vi "Actor Template-Core_Process.vi"(0 "FTW Actor Instance Configuration":string="{\n  \"Identity\": \"ActorName\",\n  \"InboxAddress\": \"tcp://127.0.0.1:*\",\n  \"PublisherAddress\": \"tcp://127.0.0.1:*\",\n  \"DebugEnableInboxLogging\": false,\n  \"DebugEnableJobLogging\": false,\n  \"DebugShowPanel\": false\n}", 11 "ErrorIn":errorcluster) -> (15 "Error":errorcluster)   [LabVIEW 2013, in "Actor Template-Core.lvclass"]
uses:
  Actor Template-Core.lvclass
  src/Instance/FTW-ActorInstance.lvclass
  src/Message/Request/FTW-Message-IncomingRequest.lvclass
panel:
  # "#TODO\nhide controls for a GUI"
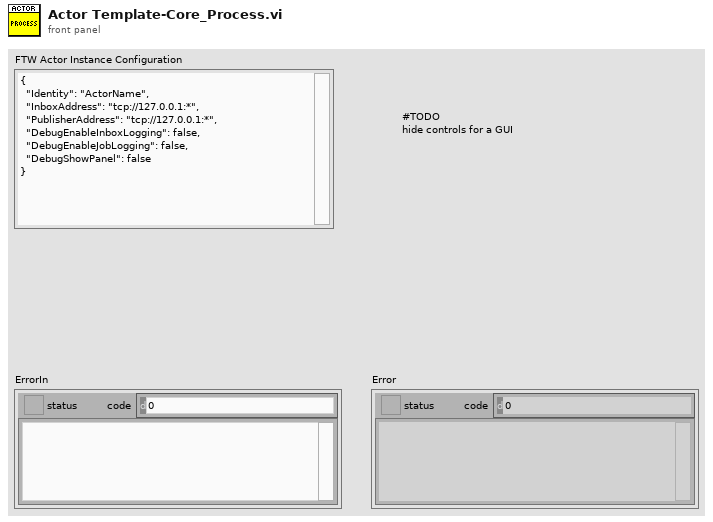
[diagram p1: front panel]
types:
  T1 = cluster{"Incoming Requests":refnum<event-registration>, "Additional Registration Types":refnum<event-registration>}
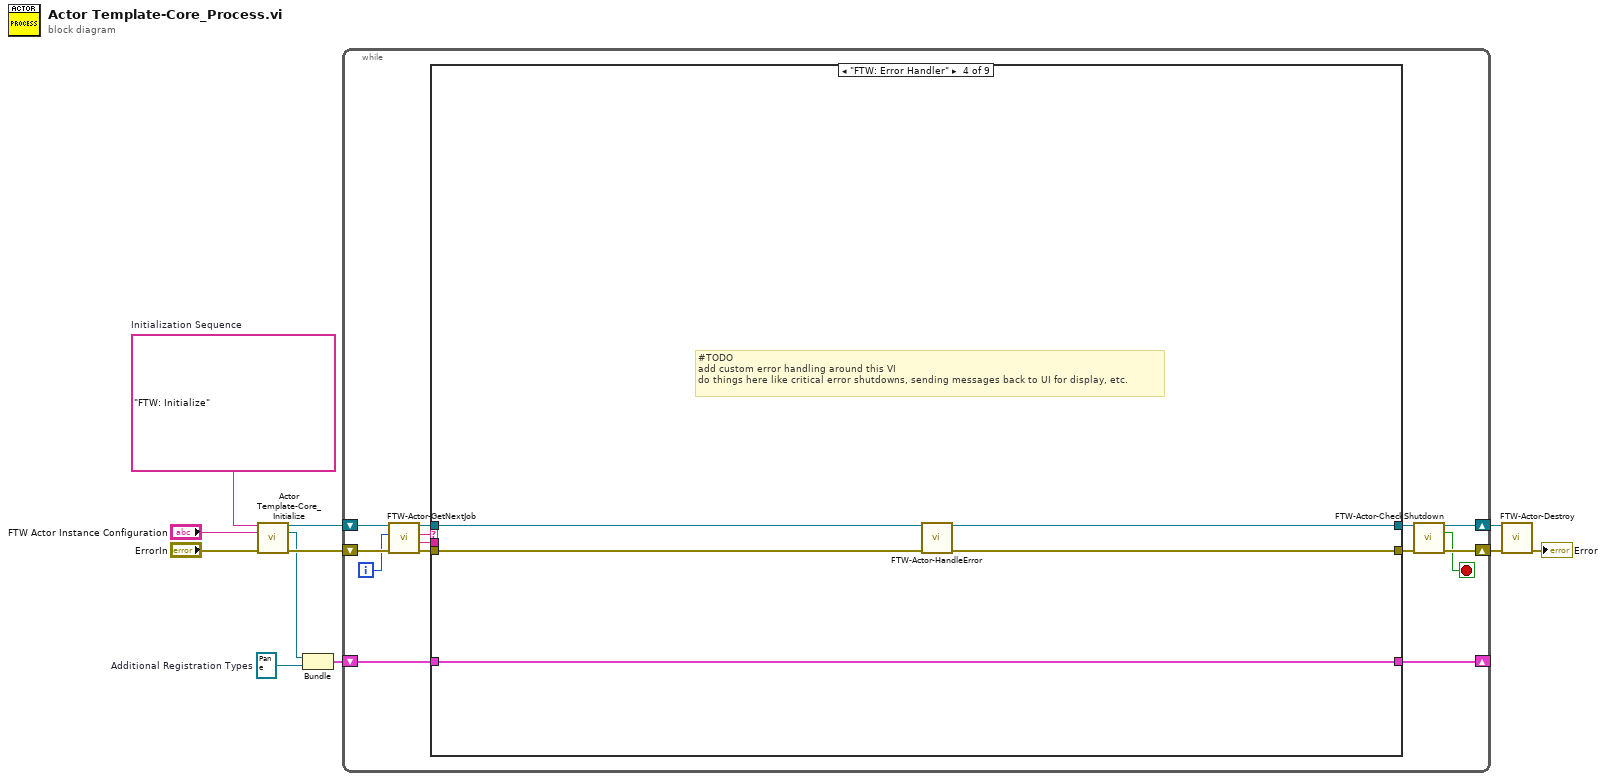
[diagram p0: block diagram]
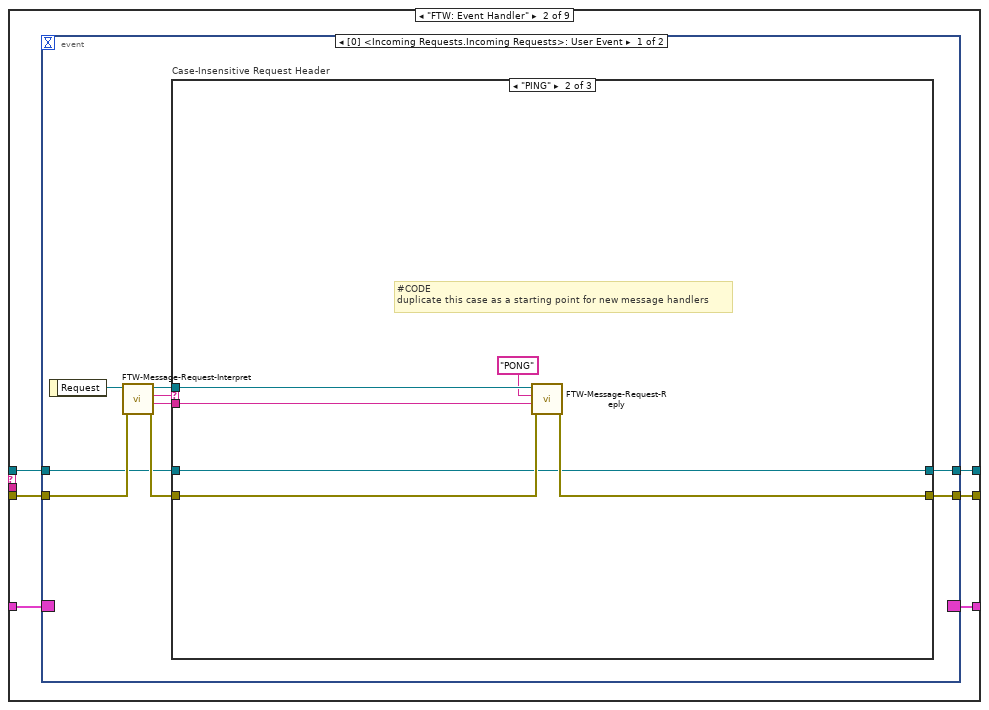
[diagram p3: hidden frame]
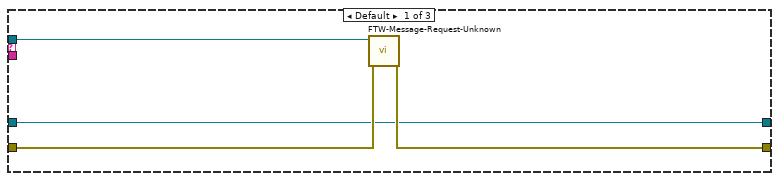
[diagram p4: hidden frame]
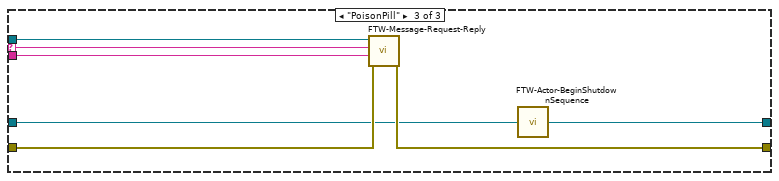
[diagram p5: hidden frame]
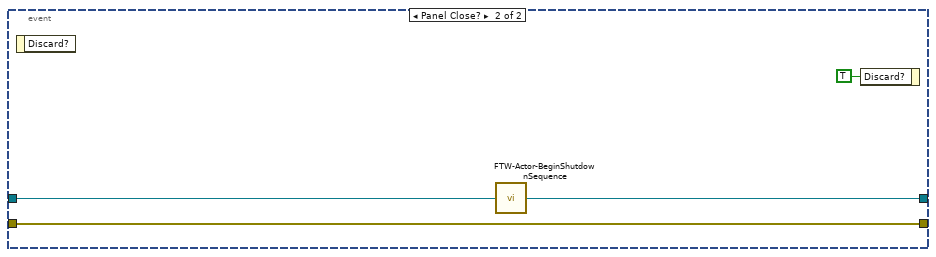
[diagram p6: hidden frame]
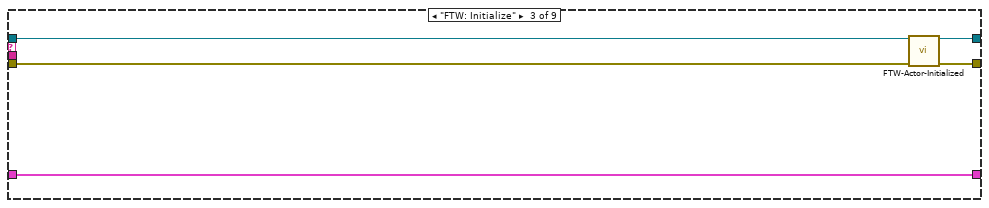
[diagram p7: hidden frame]
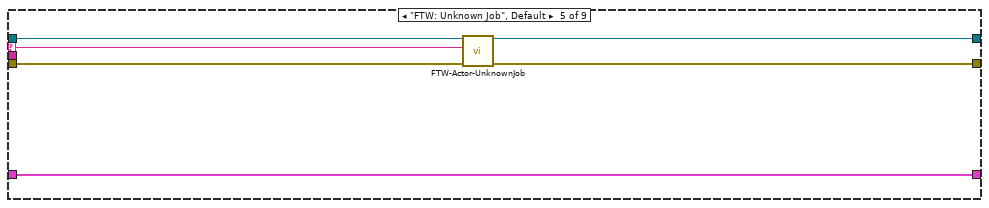
[diagram p8: hidden frame]
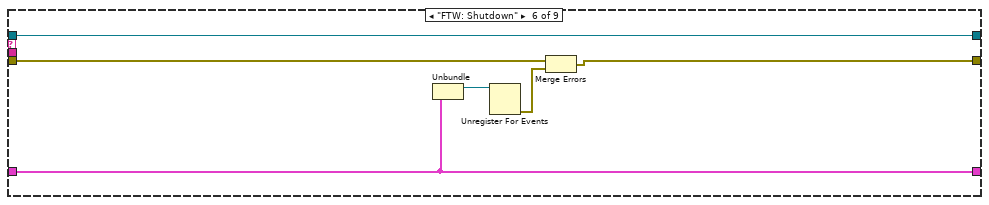
[diagram p9: hidden frame]
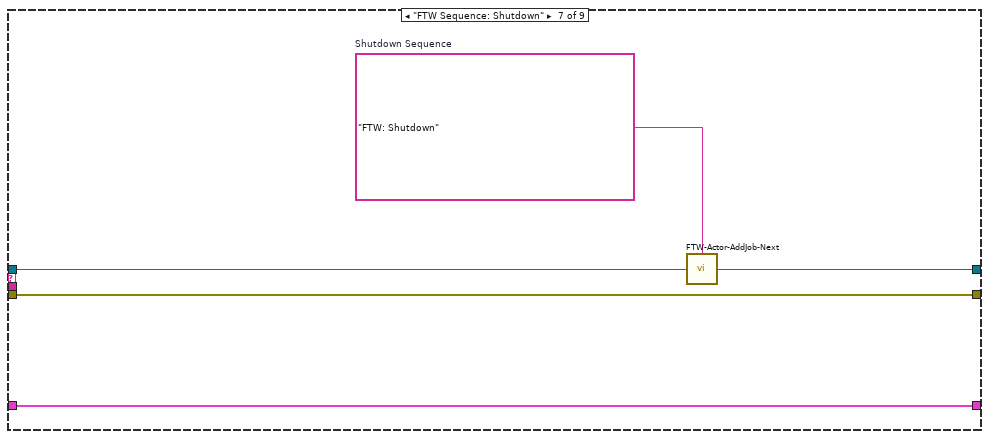
[diagram p10: hidden frame]
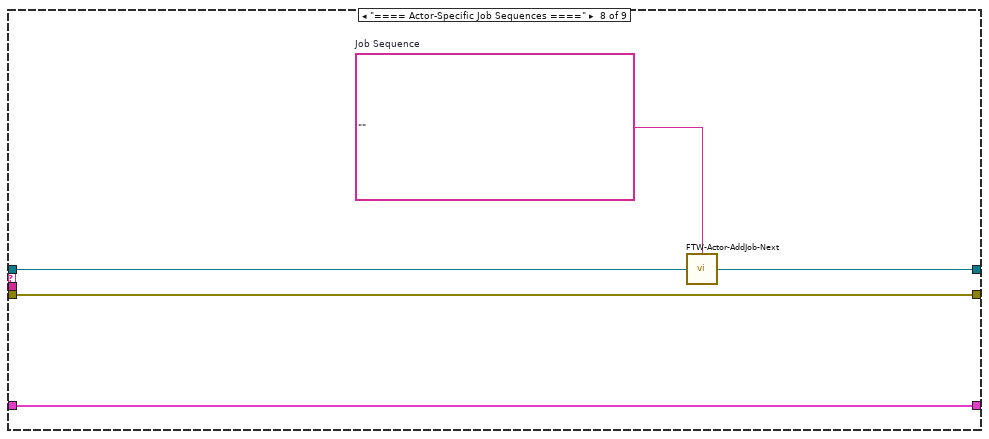
[diagram p11: hidden frame]
diagram:
  w4 = refnum<event-registration> refnum  # Additional Registration Types
  w6 = "FTW: Initialize"  # Initialization Sequence
  n1 = call "Actor Template-Core_Initialize.vi"("Initialization Sequence"=w6, "FTW Actor Instance Configuration"="FTW Actor Instance Configuration", "error in (no error)"="ErrorIn") -> ("Actor Template-Core out"=w11:refnum<class "Actor Template-Core.lvclass">, "Incoming Requests"=w1:refnum<event-registration>, "error out"=w7:errorcluster)  [unwired: 10 in]
  n2 = Bundle("Incoming Requests"=w1, "Additional Registration Types"=w4) -> (w3:T1)  [unwired: 1 in]
  n3 = while {
    shift-right: [w15] -> w9
    shift-left: w7 -> [w22]
    shift-right: [w12] -> _
    shift-left: w3 -> [w25]
    shift-right: [w17] -> w10
    shift-left: w11 -> [w24]
    i -> [w13]
    stop <- w14 stop-if-true
    n4 = call "FTW-Actor-GetNextJob.vi"("error in"=w22, "Jobs Performed"=w13, "FTW Actor Instance"=w24) -> ("error out"=w21:errorcluster, "Job Data"=w19:string, "Job Name"=w20:string, "FTW Actor Instance out"=w23:refnum<class "Actor Template-Core.lvclass">)  [unwired: 5 in]
    n5 = case shown="\"FTW: Error Handler\"" w20 {
      selector: w20 -> [_ _ _ _ w75 _ _ _ _]
      tunnel: [w27 w34 w65 w70 w78 w83 w90 w95 w99] -> w16
      tunnel: w21 -> [w27 w33 w68 w72 w79 w84 w90 w95 w99]
      tunnel: w25 -> [w28 w29 w69 w74 w80 w86 w91 w96 w98]
      tunnel: [w28 w32 w69 w74 w80 w86 w91 w96 w98] -> w12
      tunnel: w19 -> [_ _ _ _ _ _ _ _ _]
      tunnel: [w26 w31 w66 w71 w76 w81 w88 w93 w97] -> w18
      tunnel: w23 -> [w26 w30 w67 w73 w77 w81 w89 w94 w97]
      frame "==== Featherweight Framework Jobs ====" {
      }
      frame "FTW: Event Handler" {
        n6 = event shown="[0] <Incoming Requests.Incoming Requests>: User Event" {
          selector: w29 -> [_ _]
          dyn-events: [_ _] -> w32
          timeout: _ -> [_ _]
          tunnel: [w40 w63] -> w34
          tunnel: w33 -> [w41 w63]
          tunnel: [w39 w61] -> w31
          tunnel: w30 -> [w38 w62]
          event User Event {
            n7 = event-data() -> ("Request"=w42:refnum<class "FTW-Message-IncomingRequest.lvclass">)  [unwired: 1 in]
            n8 = call "FTW-Message-Request-Interpret.vi"("error in"=w41, "FTW Incoming Request"=w42) -> ("error out"=w43:errorcluster, "Request Body"=w36:string, "Request Header"=w37:string, "FTW Incoming Request out"=w35:refnum<class "FTW-Message-IncomingRequest.lvclass">)  [unwired: 6 in]
            n9 = case "Case-Insensitive Request Header" shown="\"PING\"" w37 {
              selector: w37 -> [_ _ w55]
              tunnel: [w46 w50 w57] -> w40
              tunnel: w43 -> [w47 w51 w58]
              tunnel: [w44 w48 w60] -> w39
              tunnel: w38 -> [w44 w48 w56]
              tunnel: w36 -> [_ w52 w54]
              tunnel: w35 -> [w45 w53 w59]
              frame Default {
                n10 = call "FTW-Message-Request-Unknown.vi"("error in"=w47, "FTW Incoming Request"=w45) -> ("error out"=w46:errorcluster)  [unwired: 9 in]
              }
              frame "PING" {
                # "#CODE\nduplicate this case as a starting point for new message handlers"
                n11 = call "FTW-Message-Request-Reply.vi"("error in"=w51, "Response Body"=w52, "Response Header"="PONG", "FTW Incoming Request"=w53) -> ("error out"=w50:errorcluster)  [unwired: 6 in, 1 out]
              }
              frame "PoisonPill" {
                n12 = call "FTW-Message-Request-Reply.vi"("error in"=w58, "Response Body"=w54, "Response Header"=w55, "FTW Incoming Request"=w59) -> ("error out"=w57:errorcluster)  [unwired: 6 in, 1 out]
                n13 = call "FTW-Actor-BeginShutdownSequence.vi"("FTW Actor Instance"=w56) -> ("FTW Actor Instance out"=w60:refnum<class "Actor Template-Core.lvclass">)  [unwired: 3 in]
              }
            }
          }
          event Panel Close? {
            n14 = event-data() -> ()  [unwired: 1 in, 1 out]
            n15 = call "FTW-Actor-BeginShutdownSequence.vi"("FTW Actor Instance"=w62) -> ("FTW Actor Instance out"=w61:refnum<class "Actor Template-Core.lvclass">)  [unwired: 3 in]
            n16 = event-data("Discard?"=TRUE) -> ()  [unwired: 1 in, 1 out]
          }
        }
      }
      frame "FTW: Initialize" {
        n17 = call-dynamic "FTW-Actor-Initialized.vi"("FTW Actor Instance"=w67, "error in"=w68) -> ("FTW Actor Instance out"=w66:refnum<class "Actor Template-Core.lvclass">, "error out"=w65:errorcluster)  [unwired: 12 in]
      }
      frame "FTW: Error Handler" {
        # "#TODO\nadd custom error handling around this VI\ndo things here like critical error shutdowns, sending messages back to UI for display, etc."
        n18 = call-dynamic "FTW-Actor-HandleError.vi"("FTW Actor Instance"=w73, "error in"=w72) -> ("FTW Actor Instance out"=w71:refnum<class "Actor Template-Core.lvclass">, "error out"=w70:errorcluster)  [unwired: 11 in, 1 out]
      }
      frame "FTW: Unknown Job", Default {
        n19 = call-dynamic "FTW-Actor-UnknownJob.vi"("FTW Actor Instance"=w77, "Unknown Job"=w75, "error in"=w79) -> ("FTW Actor Instance out"=w76:refnum<class "Actor Template-Core.lvclass">, "error out"=w78:errorcluster)  [unwired: 11 in]
      }
      frame "FTW: Shutdown" {
        n20 = Unbundle(w86) -> ("Incoming Requests"=w85:refnum<event-registration>)  [unwired: 1 out]
        n21 = Unregister For Events(event registration refnum=w85) -> (error out=w82:errorcluster)  [unwired: 1 in]
        n22 = Merge Errors(w84, w82) -> (w83:errorcluster)
      }
      frame "FTW Sequence: Shutdown" {
        w87 = "FTW: Shutdown"  # Shutdown Sequence
        n23 = call "FTW-Actor-AddJob-Next.vi"("Add Next in Job Queue"=w87, "FTW Actor Instance"=w89) -> ("FTW Actor Instance out"=w88:refnum<class "Actor Template-Core.lvclass">)  [unwired: 2 in]
      }
      frame "==== Actor-Specific Job Sequences ====" {
        w92 = ""  # Job Sequence
        n24 = call "FTW-Actor-AddJob-Next.vi"("Add Next in Job Queue"=w92, "FTW Actor Instance"=w94) -> ("FTW Actor Instance out"=w93:refnum<class "Actor Template-Core.lvclass">)  [unwired: 2 in]
      }
      frame "==== Actor-Specific Jobs ====" {
      }
    }
    n25 = call "FTW-Actor-CheckShutdown.vi"("FTW Actor Instance"=w18, "error in"=w16) -> ("FTW Actor Instance out"=w17:refnum<class "Actor Template-Core.lvclass">, "Shutdown?"=w14:bool, "error out"=w15:errorcluster)  [unwired: 11 in]
  }
  n26 = call-dynamic "FTW-Actor-Destroy.vi"("FTW Actor Instance"=w10, "error in"=w9) -> ("error out"=→"Error":errorcluster)  [unwired: 13 in]
